vi "Initialize.vi"(8 "error in":errorcluster, 11 "Pump Calibration Config in":T1={"Settings"={"Cycle Period"=500.0, "Ismatech"={"VISA resource name"="", "Simulated?"=TRUE, "Pump Number"=1.0, "Reverse?"=FALSE}, "Masterflex"={"VISA resource name"="", "Simulated?"=TRUE, "Pump Number"=1.0, "Reverse?"=FALSE}, "Bronkhorst M13 Flow Meter"={"VISA resource name"="", "Simulated?"=TRUE}, "PID 2 Parameters"={"Input Device"=enum."Default", "Output Device"=enum."Default"}, "Bronkhorst M14"={"VISA resource name"="", "Simulated?"=FALSE}, "Tacmina Settings"={"Analog DAQ Task"="", "Digital DAQ Task"=""}, "KNF SIMDOS Settings"={"VISA resource name"="", "Simulated?"=TRUE}, "VICI M50 Settings"={"VISA resource name"="", "Simulated?"=TRUE, "Pump Letter"="", "Reverse?"=FALSE}, "FLOM Settings"={"VISA resource name"="", "Simulated?"=TRUE, "Pump Number"=0.0}, "Calibration Limits"={"Minimum (ml/min)"=0.0, "Maximum (ml/min)"=0.0, "Steps"=0.0}, "SSI PR Settings"={"VISA resource name"="", "Simulated?"=FALSE}}, "Flowmeter Output"=0.0, "Density"=0.0, "FL Temp"=0.0, "Speed %"=0.0, "File Refnum"=refnum, "Pump On?"=enum."Not Initialized"} {"Settings"."Masterflex"."Pump Number" min=1.0 max=20.0 step=1.0; "Settings"."Ismatech"."Pump Number" min=1.0 max=20.0 step=1.0}) -> (0 "error out":errorcluster, 3 "Pump Calibration Config Out":T1={"Settings"={"Cycle Period"=500.0, "Ismatech"={"VISA resource name"="", "Simulated?"=TRUE, "Pump Number"=1.0, "Reverse?"=FALSE}, "Masterflex"={"VISA resource name"="", "Simulated?"=TRUE, "Pump Number"=1.0, "Reverse?"=FALSE}, "Bronkhorst M13 Flow Meter"={"VISA resource name"="", "Simulated?"=TRUE}, "PID 2 Parameters"={"Input Device"=enum."Default", "Output Device"=enum."Default"}, "Bronkhorst M14"={"VISA resource name"="", "Simulated?"=FALSE}, "Tacmina Settings"={"Analog DAQ Task"="", "Digital DAQ Task"=""}, "KNF SIMDOS Settings"={"VISA resource name"="", "Simulated?"=TRUE}, "VICI M50 Settings"={"VISA resource name"="", "Simulated?"=TRUE, "Pump Letter"="", "Reverse?"=FALSE}, "FLOM Settings"={"VISA resource name"="", "Simulated?"=TRUE, "Pump Number"=0.0}, "Calibration Limits"={"Minimum (ml/min)"=0.0, "Maximum (ml/min)"=0.0, "Steps"=0.0}, "SSI PR Settings"={"VISA resource name"="", "Simulated?"=FALSE}}, "Flowmeter Output"=0.0, "Density"=0.0, "FL Temp"=0.0, "Speed %"=0.0, "File Refnum"=refnum, "Pump On?"=enum."Not Initialized"} {"Settings"."Masterflex"."Pump Number" min=1.0 max=20.0 step=1.0; "Settings"."Ismatech"."Pump Number" min=1.0 max=20.0 step=1.0})   [LabVIEW 2018, in "Calibration.lvlib" / "Engine.lvlib"]
uses:
  Engine.lvlib
  Pump Calibration Config.ctl
  Pfizer Timed Seq/Software/Ismatec ISM 831C/Controls/Ismatech Settings Cluster.ctl
  Pfizer Timed Seq/Software/Masterflex 7550-30/Controls/Settings Cluster.ctl
  Pfizer Timed Seq/Software/Bronkhorst M13 Flow Meter/Settings Cluster.ctl
  Pfizer Timed Seq/Software/Measure Instrument/PID Input Enum.ctl
  Pfizer Timed Seq/Software/Measure Instrument/PID 2 Output Enum.ctl
  Pfizer Timed Seq/Software/Mettler Toledo/Controls/Settings Cluster.ctl
  Pfizer Timed Seq/Software/Tacmina QI/Tacmina QI DAQ Setting.ctl
  Pfizer Timed Seq/Software/KNF Pump/Settings Cluster plus SIMDOS.ctl
  Pfizer Timed Seq/Software/VICI M50 Party Mode/Settings Cluster.ctl
  Pfizer Timed Seq/Software/FLOM Pump/Settings Cluster.ctl
  Pfizer Timed Seq/Software/SSI PR Class/SSI PR or LD Settings Cluster.ctl
  Pfizer Timed Seq/Software/Bronkhorst M13 Flow Meter/Bronkhorst M13 Flow Meter.lvlib
  Pfizer Timed Seq/Software/Bronkhorst M14 Flow Meter/Bronkhorst M14 Flow Meter.lvlib
  Pfizer Timed Seq/Software/Ismatec ISM 831C/Ismatec ISM 831C.lvlib
  Pfizer Timed Seq/Software/Masterflex 7550-30/Masterflex 7550-30.lvlib
  Pfizer Timed Seq/Software/VICI M50 Party Mode/VICI M6 M50 Party Mode.lvlib
  Pfizer Timed Seq/Software/Tacmina QI/Tacmina QI.lvlib
  Pfizer Timed Seq/Software/KNF Pump/KNF SIMDOS.lvlib
  Pfizer Timed Seq/Software/FLOM Pump/FLOM Pump.lvlib
  Pfizer Timed Seq/Software/Mettler Toledo/Mettler Toledo.lvlib
  Pfizer Timed Seq/Software/Calibration VIs/Calibration.lvlib
  Pfizer Timed Seq/Software/SSI PR Class/SSI PR or LD Pump.lvlib
panel:
  # "Output Instruments"
  # "Input Instruments"
  # "Output Instruments"
  # "Input Instruments"
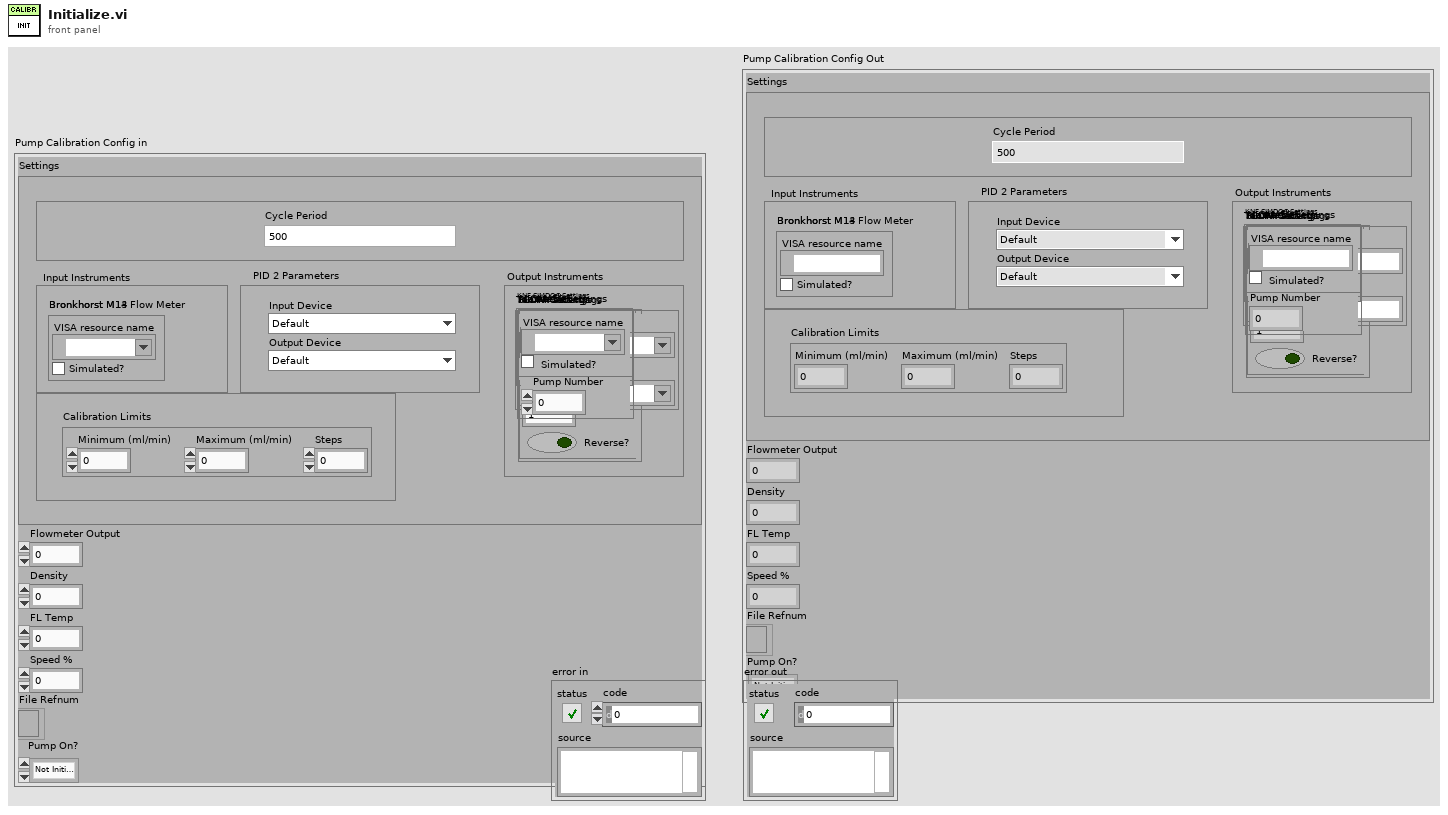
[diagram p1: front panel]
types:
  T1 = typedef "Calibration.lvlib/Pump Calibration Config.ctl" = cluster{"Settings":cluster{"Cycle Period":dbl, "Ismatech":T2, "Masterflex":T3, "Bronkhorst M13 Flow Meter":T4, "PID 2 Parameters":cluster{"Input Device":T5, "Output Device":T6}, "Bronkhorst M14":T7, "Tacmina Settings":T8, "KNF SIMDOS Settings":T9, "VICI M50 Settings":T10, "FLOM Settings":T11, "Calibration Limits":cluster{"Minimum (ml/min)":dbl, "Maximum (ml/min)":dbl, "Steps":dbl}, "SSI PR Settings":T12}, "Flowmeter Output":dbl, "Density":dbl, "FL Temp":dbl, "Speed %":dbl, "File Refnum":refnum<file>, "Pump On?":enum16{"Off", "On", "Not Initialized"}}
  T2 = typedef "Ismatec ISM 831C.lvlib/Ismatech Settings Cluster.ctl" = cluster{"VISA resource name":refnum<visa-resource-name>, "Simulated?":bool, "Pump Number":dbl, "Reverse?":bool}
  T3 = typedef "Masterflex 7550-30.lvlib/Settings Cluster.ctl" = cluster{"VISA resource name":refnum<visa-resource-name>, "Simulated?":bool, "Pump Number":dbl, "Reverse?":bool}
  T4 = typedef "Bronkhorst M13 Flow Meter.lvlib/Settings Cluster.ctl" = cluster{"VISA resource name":refnum<visa-resource-name>, "Simulated?":bool}
  T5 = typedef "PID Input Enum.ctl" = enum16{"Default", "Bronkhorst M13", "Bronkhorst M14", "Scale Rate of Change"}
  T6 = typedef "PID 2 Output Enum.ctl" = enum16{"Default", "Ismatec ISM 831C", "Masterflex 7550-30", "VICI", "Tacmina QI", "KNF SIMDOS", "ASIA Type C", "FLOM UI-22-11", "SSI PR", "Masterflex 75211-70"}
  T7 = typedef "Mettler Toledo.lvlib/Settings Cluster.ctl" = cluster{"VISA resource name":refnum<visa-resource-name>, "Simulated?":bool}
  T8 = typedef "Tacmina QI.lvlib/Tacmina QI DAQ Setting.ctl" = cluster{"Analog DAQ Task":refnum<k21>, "Digital DAQ Task":refnum<k21>}
  T9 = typedef "KNF SIMDOS.lvlib/Settings Cluster plus SIMDOS.ctl" = cluster{"VISA resource name":refnum<visa-resource-name>, "Simulated?":bool}
  T10 = typedef "VICI M6 M50 Party Mode.lvlib/Settings Cluster.ctl" = cluster{"VISA resource name":refnum<visa-resource-name>, "Simulated?":bool, "Pump Letter":string, "Reverse?":bool}
  T11 = typedef "FLOM Pump.lvlib/Settings Cluster.ctl" = cluster{"VISA resource name":refnum<visa-resource-name>, "Simulated?":bool, "Pump Number":dbl}
  T12 = typedef "SSI PR or LD Pump.lvlib/SSI PR or LD Settings Cluster.ctl" = cluster{"VISA resource name":refnum<visa-resource-name>, "Simulated?":bool}
  T13 = cluster{"Cycle Period":dbl, "Ismatech":T2, "Masterflex":T3, "Bronkhorst M13 Flow Meter":T4, "PID 2 Parameters":cluster{"Input Device":T5, "Output Device":T6}, "Bronkhorst M14":T7, "Tacmina Settings":T8, "KNF SIMDOS Settings":T9, "VICI M50 Settings":T10, "FLOM Settings":T11, "Calibration Limits":cluster{"Minimum (ml/min)":dbl, "Maximum (ml/min)":dbl, "Steps":dbl}, "SSI PR Settings":T12}
  T14 = typedef "Bronkhorst M14 Flow Meter.lvlib/Settings Cluster.ctl" = cluster{"VISA resource name":refnum<visa-resource-name>, "Simulated?":bool}
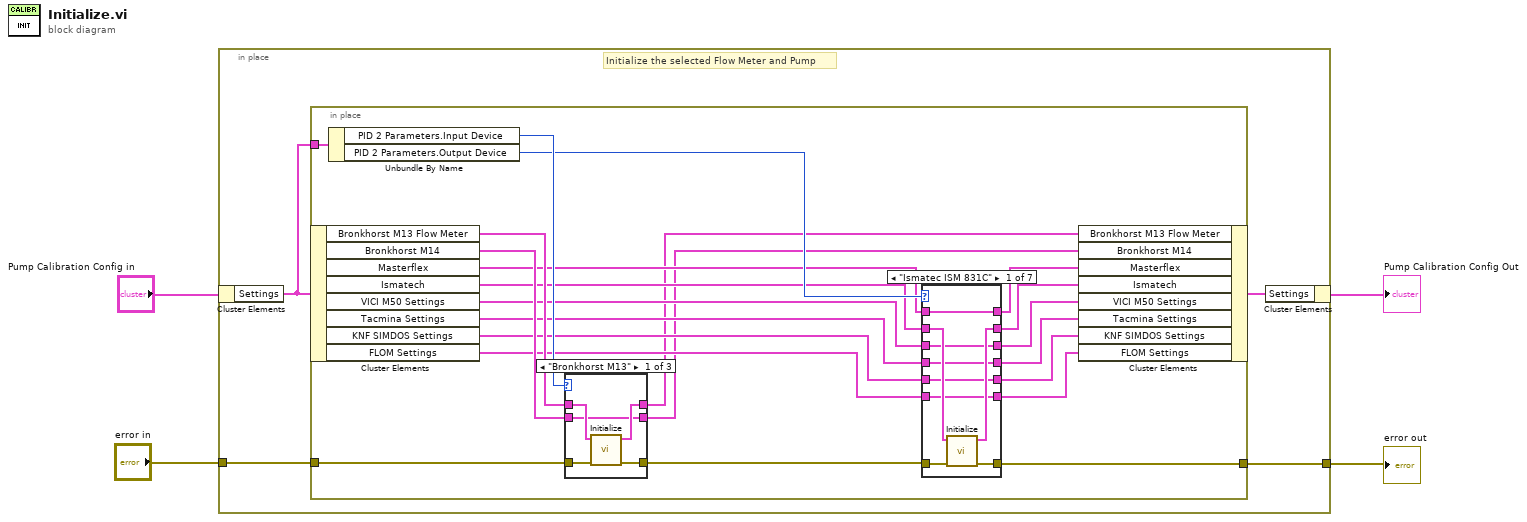
[diagram p0: block diagram]
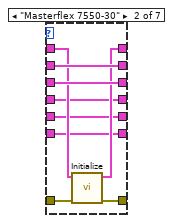
[diagram p2: hidden frame]
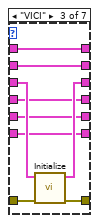
[diagram p3: hidden frame]
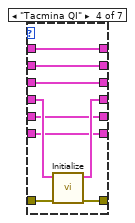
[diagram p4: hidden frame]
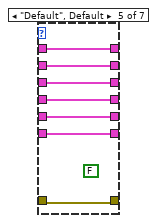
[diagram p5: hidden frame]
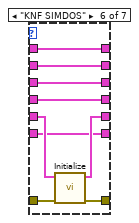
[diagram p6: hidden frame]
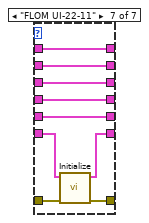
[diagram p7: hidden frame]
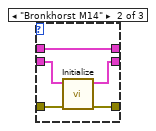
[diagram p8: hidden frame]
diagram:
  n1 = in-place {
    in-place-border: "error in" -> [w8]
    in-place-border: [w7] -> w1
    # "Initialize the selected Flow Meter and Pump"
    n2 = in-place-cluster #1("Pump Calibration Config in") -> ("Settings"=w6:T13)
    n3 = in-place {
      in-place-border: w8 -> [w30]
      in-place-border: w6 -> [w26]
      in-place-border: [w25] -> w7
      n4 = in-place-cluster #2(w6) -> ("Bronkhorst M13 Flow Meter"=w24:T4, "Bronkhorst M14"=w23:T7, "Masterflex"=w22:T3, "Ismatech"=w21:T2, "VICI M50 Settings"=w20:T10, "Tacmina Settings"=w19:T8, "KNF SIMDOS Settings"=w18:T9, "FLOM Settings"=w17:T11)
      n5 = Unbundle By Name(w26) -> ("PID 2 Parameters.Input Device"=w29:T5, "PID 2 Parameters.Output Device"=w28:T6)
      n6 = case shown="\"Bronkhorst M13\"" w29 {
        tunnel: w24 -> [w96 w99 w104]
        tunnel: w30 -> [w95 w101 w103]
        tunnel: [w94 w100 w103] -> w27
        tunnel: [w93 w99 w104] -> w16
        tunnel: w23 -> [w92 w98 w102]
        tunnel: [w92 w97 w102] -> w15
        frame "Bronkhorst M13" {
          n7 = call "Initialize.vi"("error in (no error)"=w95, "Bronkhorst Settings in"=w96) -> ("error out"=w94:errorcluster, "Bronkhorst Settings out"=w93:T4)  [unwired: 7 in, 1 out]
        }
        frame "Bronkhorst M14" {
          n8 = call "Initialize.vi"("error in (no error)"=w101, "Bronkhorst Settings in"=w98) -> ("error out"=w100:errorcluster, "Bronkhorst Settings out"=w97:T14)  [unwired: 7 in, 1 out]
        }
        frame "Default", Default {
        }
      }
      n9 = case shown="\"Ismatec ISM 831C\"" w28 {
        tunnel: w22 -> [w36 w46 w52 w63 w73 w82 w91]
        tunnel: [w36 w45 w52 w63 w73 w82 w91] -> w14
        tunnel: w27 -> [w39 w43 w54 w65 w71 w78 w86]
        tunnel: [w35 w44 w55 w66 w71 w77 w85] -> w25
        tunnel: w21 -> [w38 w48 w53 w64 w72 w81 w90]
        tunnel: [w37 w48 w53 w64 w72 w81 w90] -> w13
        tunnel: w20 -> [w34 w47 w57 w62 w69 w80 w89]
        tunnel: [w34 w47 w56 w62 w69 w80 w89] -> w12
        tunnel: w19 -> [w33 w42 w51 w61 w70 w79 w88]
        tunnel: [w33 w42 w51 w60 w70 w79 w88] -> w11
        tunnel: w18 -> [w32 w41 w50 w59 w68 w75 w87]
        tunnel: [w32 w41 w50 w59 w68 w76 w87] -> w10
        tunnel: w17 -> [w31 w40 w49 w58 w67 w74 w83]
        tunnel: [w31 w40 w49 w58 w67 w74 w84] -> w9
        frame "Ismatec ISM 831C" {
          n10 = call "Initialize.vi"("error in (no error)"=w39, "Ismatech Settings"=w38) -> ("error out"=w35:errorcluster, "Ismatech Settings"=w37:T2)  [unwired: 6 in, 2 out]
        }
        frame "Masterflex 7550-30" {
          n11 = call "Initialize.vi"("error in (no error)"=w43, "Masterflex Settings in"=w46) -> ("error out"=w44:errorcluster, "Masterflex Settings out"=w45:T3)  [unwired: 6 in, 2 out]
        }
        frame "VICI" {
          n12 = call "Initialize.vi"("error in (no error)"=w54, "VICI Settings"=w57) -> ("error out"=w55:errorcluster, "VICI Settings"=w56:T10)  [unwired: 6 in, 2 out]
        }
        frame "Tacmina QI" {
          n13 = call "Initialize.vi"("error in"=w65, "Tacmina Settings in"=w61) -> ("error out"=w66:errorcluster, "Tacmina Settings out"=w60:T8)  [unwired: 7 in, 1 out]
        }
        frame "Default", Default {
          (unwired) FALSE ("Initialized")
        }
        frame "KNF SIMDOS" {
          n14 = call "Initialize.vi"("error in (no error)"=w78, "KNF Settings In"=w75) -> ("error IO"=w77:errorcluster, "KNF Settings Out"=w76:T9)  [unwired: 6 in, 2 out]
        }
        frame "FLOM UI-22-11" {
          n15 = call "Initialize.vi"("error in (no error)"=w86, "FLOM Settings in"=w83) -> ("error out"=w85:errorcluster, "FLOM Settings out"=w84:T11)  [unwired: 6 in, 2 out]
        }
      }
      n16 = in-place-cluster #2("Bronkhorst M13 Flow Meter"=w16, "Bronkhorst M14"=w15, "Masterflex"=w14, "Ismatech"=w13, "VICI M50 Settings"=w12, "Tacmina Settings"=w11, "KNF SIMDOS Settings"=w10, "FLOM Settings"=w9) -> (w5:T13)
    }
    n17 = in-place-cluster #1("Settings"=w5) -> (→"Pump Calibration Config Out":T1)
  }
  "error out" <- w1
